vi "Add Remove Test.vi"() -> (0 "error out":errorcluster, 2 "Success Delete":bool, 3 "Success ADD":bool)   [LabVIEW 2014, in "DAQmx Module Tests.lvlib"]
doc: "Tests the Add Line and Remove Line functions."
uses:
  DAQmx Module Tests.lvlib
  module/configuration/Line.ctl
  <vilib>/NI/Tag Bus Module Framework/channel/TBM channel.lvclass
  module/configuration/Measurement Type.ctl
  module/configuration/Parameters.ctl
  module/configuration/DAQmx Module Configuration.lvclass
  editor node/DAQmx Module Editor Node.lvclass
panel:
  out "Deleted Line":string
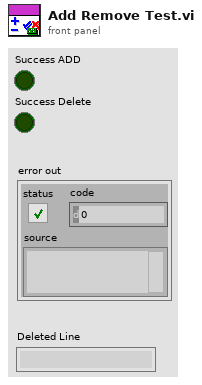
[diagram p1: front panel]
types:
  T1 = typedef "DAQmx Module Configuration.lvclass/Measurement Type.ctl" = enum16{"Digital Input", "Digital Output", "Voltage Input", "Voltage Output", "Current Input", "Current Output", "RTD", "Thermocouple", "Strain"}
  T2 = typedef "Daqmx Module configuration.lvclass/Line.ctl" = cluster{"channel":refnum<class "TBM channel.lvclass">, "Physical Channel":string, "Measurement Type":T3, "Parameters":T4}
  T3 = typedef "Daqmx Module configuration.lvclass/Measurement Type.ctl" = enum16{"Digital Input", "Digital Output", "Voltage Input", "Voltage Output", "Current Input", "Current Output", "RTD", "Thermocouple", "Strain"}
  T4 = typedef "Daqmx Module configuration.lvclass/Parameters.ctl" = cluster{"Digital Config":cluster{"Invert Lines?":bool}, "Voltage Config":cluster{"Maximum Value (V)":dbl, "Minimum Value (V)":dbl, "in terminal configuration (V)":i32, "out terminal configuration (V)":i32}, "Current Config":cluster{"Maximum Value (A)":dbl, "Minimum Value (A)":dbl, "shunt resistor location":i32, "input terminal configuration (C)":i32, "external shunt resistor value":dbl}, "RTD Config":cluster{"Maximum Value (°C)":dbl, "Minimum Value (°C)":dbl, "resistance configuration":i32, "r0":dbl, "current excitation value":dbl, "rtd type":i32, "current excitation source":i32}, "Thermocouple Config":cluster{"Minimum Value (C)":dbl, "Maximum Value (C)":dbl, "thermocouple type":i32, "cjc source":i32, "cjc value":dbl}, "Strain Config":cluster{"Maximum Value":dbl, "Minimum Value":dbl, "bridge information":cluster{"strain configuration":i32, "lead wire resistance":dbl, "initial bridge voltage":dbl, "voltage excitation source":i32, "voltage excitation value":dbl}, "strain gage information":cluster{"gage factor":dbl, "nominal gage resistance":dbl, "poisson ratio":dbl}}}
  T5 = typedef "TBM channel.lvclass/channel classification.ctl" = enum16{"input data", "output data", "processing parameter", "processing result"}
  T6 = typedef "tag bus.lvlib/tag descriptor.lvclass/Data Type.ctl" = enum16{"Double", "Single", "I64", "I32", "I16", "I8", "U64", "U32", "U16", "U8", "Boolean", "String", "Array of Double", "Array of Single", "Array of I64", "Array of I32", "Array of I16", "Array of I8", "Array of U64", "Array of U32", "Array of U16", "Array of U8", "Array of Boolean", "Array of String"}
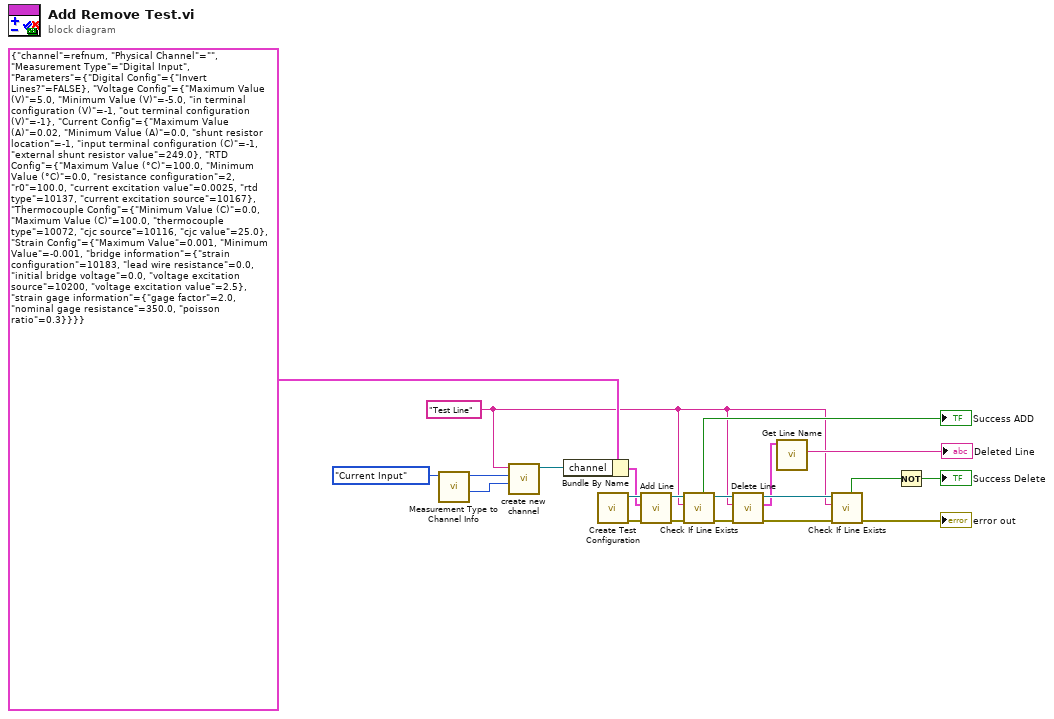
[diagram p0: block diagram]
diagram:
  w4 = "Test Line" ("channel name")
  n1 = call "Measurement Type to Channel Info.vi"("Measurement Type"=Measurement_Type."Current Input") -> ("channel classification"=w2:T5, "Data Type"=w3:T6)  [unwired: 8 in]
  n2 = call <vilib>:"create new channel.vi"("channel classification"=w2, "data type"=w3, "channel name"=w4) -> ("channel"=w20:refnum<class "TBM channel.lvclass">)  [unwired: 8 in]
  n3 = Bundle By Name(cluster=T2 {"channel"=refnum, "Physical Channel"="", "Measurement Type"=enum."Digital Input", "Parameters"={"Digital Config"={"Invert Lines?"=FALSE}, "Voltage Config"={"Maximum Value (V)"=5.0, "Minimum Value (V)"=-5.0, "in terminal configuration (V)"=-1, "out terminal configuration (V)"=-1}, "Current Config"={"Maximum Value (A)"=0.02, "Minimum Value (A)"=0.0, "shunt resistor location"=-1, "input terminal configuration (C)"=-1, "external shunt resistor value"=249.0}, "RTD Config"={"Maximum Value (°C)"=100.0, "Minimum Value (°C)"=0.0, "resistance configuration"=2, "r0"=100.0, "current excitation value"=0.0025, "rtd type"=10137, "current excitation source"=10167}, "Thermocouple Config"={"Minimum Value (C)"=0.0, "Maximum Value (C)"=100.0, "thermocouple type"=10072, "cjc source"=10116, "cjc value"=25.0}, "Strain Config"={"Maximum Value"=0.001, "Minimum Value"=-0.001, "bridge information"={"strain configuration"=10183, "lead wire resistance"=0.0, "initial bridge voltage"=0.0, "voltage excitation source"=10200, "voltage excitation value"=2.5}, "strain gage information"={"gage factor"=2.0, "nominal gage resistance"=350.0, "poisson ratio"=0.3}}}} ("Line"), "channel"=w20) -> (w18:T2)
  n4 = call "Create Test Configuration.vi"() -> ("error out"=w12:errorcluster, "Module Configuration"=w21:refnum<class "DAQmx Module Configuration.lvclass">)  [unwired: 6 in, 4 out]
  n5 = call "Add Line.vi"("error in"=w12, "Line"=w18, "Daqmx Module configuration in"=w21) -> ("error out"=w14:errorcluster, "Daqmx Module configuration out"=w17:refnum<class "DAQmx Module Configuration.lvclass">)  [unwired: 6 in, 1 out]
  n6 = call-dynamic "Check If Line Exists.vi"("error in"=w14, "Name to Locate"=w4, "Daqmx Module configuration in"=w17) -> ("error out"=w13:errorcluster, "Daqmx Module configuration out"=w16:refnum<class "DAQmx Module Configuration.lvclass">, "Found?"=→"Success ADD":bool)  [unwired: 4 in, 2 out]
  n7 = call "Delete Line.vi"("error in"=w13, "Line Name"=w4, "Daqmx Module configuration in"=w16) -> ("error out"=w11:errorcluster, "Deleted Line"=w6:T2, "Daqmx Module configuration out"=w9:refnum<class "DAQmx Module Configuration.lvclass">)  [unwired: 6 in]
  n8 = call "Get Line Name.vi"("Line in"=w6) -> ("Name"=→"Deleted Line":string)  [unwired: 8 in, 2 out]
  n9 = call-dynamic "Check If Line Exists.vi"("error in"=w11, "Name to Locate"=w4, "Daqmx Module configuration in"=w9) -> ("error out"=→"error out":errorcluster, "Found?"=w8:bool)  [unwired: 4 in, 3 out]
  n10 = Not(x=w8) -> (.not. x?=→"Success Delete":bool)
